vi "TestHemisphere.vi"() -> ()   [LabVIEW 2013]
uses:
  Data/TypeDefs/UTM Location.ctl
  <vilib>/myRIO/Common/Instrument Driver Framework/myRIO v1.0/UART/vis/myRIO v1.0 Close UART.vi
  <vilib>/myRIO/Common/Instrument Driver Framework/Utilities/vis/FPGA Ref Manager.vi
  <vilib>/myRIO/Common/Instrument Driver Framework/myRIO v1.0/myRIO v1.0 Reset FPGA.vi
  <vilib>/myRIO/Instrument Drivers/Utilities/Utilities.lvlib
panel:
  out "Serial Settings:Baud Rate":u32
  out "Raw string":string
  out "VISA read buffer":string
  out "Stop  Button\nHeartbeat":bool
  out "Stop Button\nLoop modulo":i32
  out "Read loop counter":i32
  out "Heartbeat":bool
  out "Roll":dbl
  out "Pitch":dbl
  out "Boat Speed":dbl
  out "Boat Direction":dbl
  out "Boat Location":T1 {"North" format="%#_10f"; "East" format="%#_8f"}
  in  "stop":bool
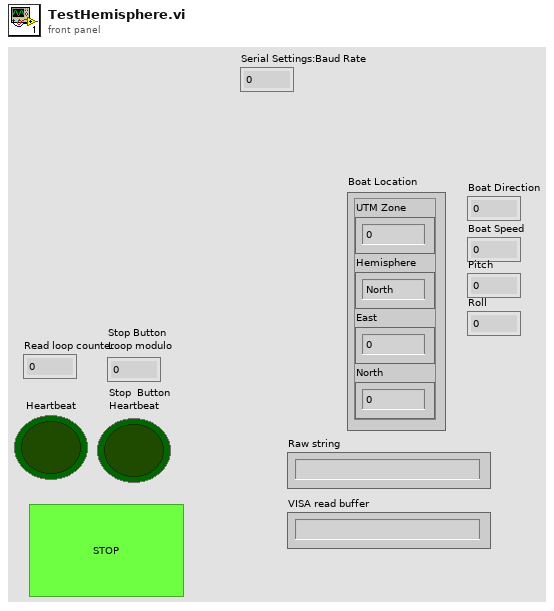
[diagram p1: front panel]
types:
  T1 = typedef "UTM Location.ctl" = cluster{"UTM Zone":dbl, "Hemisphere":enum16{"North", "South"}, "East":dbl, "North":dbl}
  T2 = typedef "Notifiers.ctl" = cluster{"BoatSpeed":refnum<notifier>, "WindSpeed":refnum<notifier>, "MissionCheckOff":refnum<notifier>, "EStop":refnum<notifier>, "SpeedOverWater":refnum<notifier>, "BoatDirection":refnum<notifier>, "Luffing":refnum<notifier>, "RudderForce":refnum<notifier>, "BatteryVoltage":refnum<notifier>, "StayForces":refnum<notifier>, "BoatLocation":refnum<notifier>, "Pitch":refnum<notifier>, "Roll":refnum<notifier>, "RateOfTurn":refnum<notifier>, "RelWindDirection":refnum<notifier>, "SailPositions":refnum<notifier>, "RudderPosition":refnum<notifier>, "IronsRange":refnum<notifier>, "AbsWindDirection":refnum<notifier>, "OverrideInformation":refnum<notifier>, "DynamixelTorques":refnum<notifier>, "MotorSetup":refnum<notifier>, "Airmar Status":refnum<notifier>, "HardwareOnline?":refnum<notifier>, "AcutalSimSailPositions":refnum<notifier>, "DynamixelCycleTracker":refnum<notifier>}
  T3 = typedef "GPS-Compass Queue Cluster.ctl" = cluster{"BoatLocation Queue":refnum<queue>, "BoatDirection Queue":refnum<queue>, "BoatSpeed Queue":refnum<queue>, "RateOfTurn Queue":refnum<queue>, "Pitch Queue":refnum<queue>, "Roll Queue":refnum<queue>}
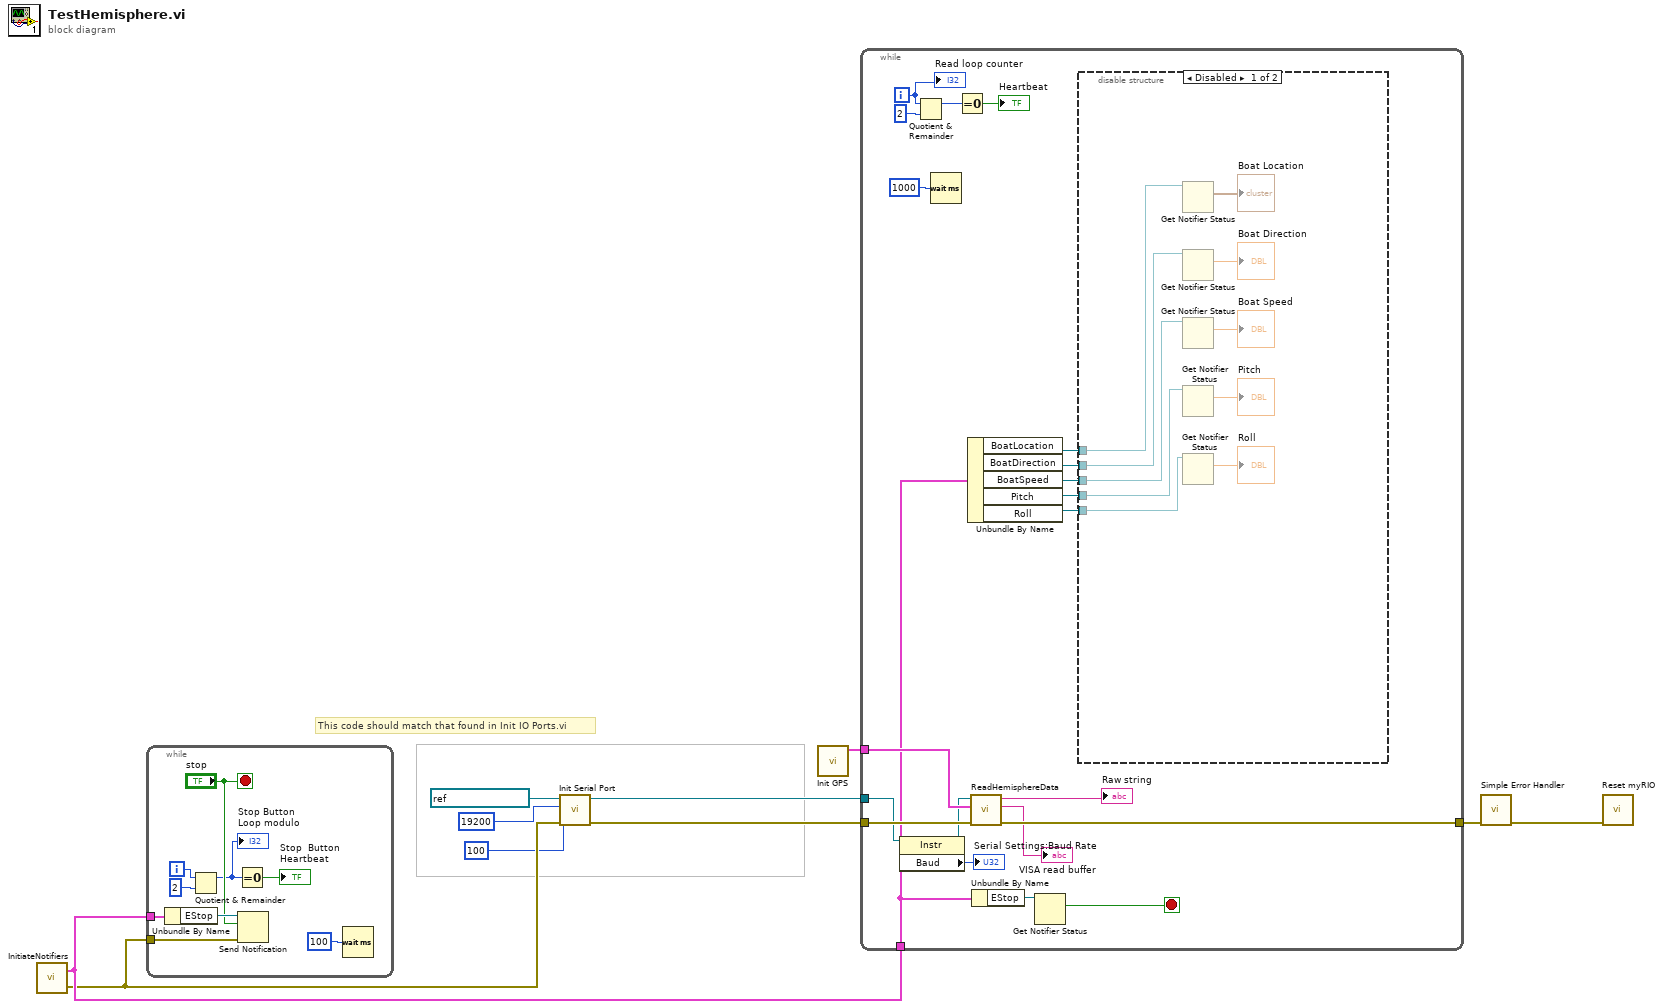
[diagram p0: block diagram]
diagram:
  # "This code should match that found in Init IO Ports.vi"
  n1 = call "InitiateNotifiers.vi"() -> ("error out"=w2:errorcluster, "NotifierReferences"=w7:T2)  [unwired: 2 in]
  n2 = while {
    tunnel: w7 -> [w17]
    tunnel: w2 -> [w11]
    i -> [w13]
    stop <- "stop" stop-if-true
    n3 = Unbundle By Name(w17) -> ("EStop"=w18:refnum<notifier>)
    n4 = Quotient & Remainder(x=w13, y=2) -> (x-y*floor(x/y)=w12:i32)  [unwired: 1 out]
    "Stop Button\nLoop modulo" <- w12
    n5 = Equal To 0?(x=w12) -> (x = 0?=→"Stop  Button\nHeartbeat":bool)
    n6 = Send Notification(notification="stop", notifier=w18, error in (no error)=w11) -> ()  [unwired: 2 out]
    n7 = Wait (ms)(milliseconds to wait=u32 100) -> ()  [unwired: 1 out]
  }
  n8 = call "Init Serial Port.vi"("error in (no error)"=w2, "Input\nbuffer size"=u32 100 ("Input\nbuffer size"), "baud rate"=u32 19200, "VISA Refnum in"=refnum<visa-resource-name> "ASRL1::INSTR") -> ("error out"=w5:errorcluster, "VISA Refnum out"=w6:refnum<visa-resource-name>)  [unwired: 6 in]
  n9 = call "Init GPS.vi"() -> ("GPS-Compass Queue Cluster"=w10:T3)  [unwired: 11 in]
  n10 = while {
    tunnel: w10 -> [w39]
    tunnel: w7 -> [w28]
    tunnel: [w31] -> w9
    tunnel: w6 -> [w23]
    tunnel: w5 -> [w29]
    i -> [w25]
    stop <- w20 stop-if-true
    n11 = property class="Instr"(reference=w23) -> (reference out=w22:refnum<visa-resource-name>, "Baud"=→"Serial Settings:Baud Rate":u32)  [unwired: 1 in, 1 out]
    n12 = Quotient & Remainder(x=w25, y=2) -> (x-y*floor(x/y)=w30:i32)  [unwired: 1 out]
    n13 = Wait (ms)(milliseconds to wait=u32 1000) -> ()  [unwired: 1 out]
    n14 = Equal To 0?(x=w30) -> (x = 0?=→"Heartbeat":bool)
    n15 = Unbundle By Name(w28) -> ("BoatLocation"=w38:refnum<notifier>, "BoatDirection"=w37:refnum<notifier>, "BoatSpeed"=w36:refnum<notifier>, "Pitch"=w35:refnum<notifier>, "Roll"=w34:refnum<notifier>)
    n16 = call "ReadHemisphereData.vi"("Error in"=w29, "Hemisphere Queue Cluster"=w39, "VISA UART port"=w22) -> ("Error out"=w31:errorcluster, "Sentence"=→"VISA read buffer":string, "Raw string"=→"Raw string":string)  [unwired: 6 in]
    n17 = Unbundle By Name(w28) -> ("EStop"=w27:refnum<notifier>)
    n18 = Get Notifier Status(notifier=w27) -> (current notification=w20:bool)  [unwired: 1 in, 4 out]
    n19 = disable-structure shown="Disabled" {
      disable-tunnel: w38 -> [w50 _]
      disable-tunnel: w37 -> [w49 _]
      disable-tunnel: w36 -> [w48 _]
      disable-tunnel: w35 -> [w47 _]
      disable-tunnel: w34 -> [w46 _]
      frame Disabled {
        n20 = Get Notifier Status(notifier=w50) -> (current notification=→"Boat Location":T1)  [unwired: 1 in, 4 out]
        n21 = Get Notifier Status(notifier=w49) -> (current notification=→"Boat Direction":dbl)  [unwired: 1 in, 4 out]
        n22 = Get Notifier Status(notifier=w48) -> (current notification=→"Boat Speed":dbl)  [unwired: 1 in, 4 out]
        n23 = Get Notifier Status(notifier=w47) -> (current notification=→"Pitch":dbl)  [unwired: 1 in, 4 out]
        n24 = Get Notifier Status(notifier=w46) -> (current notification=→"Roll":dbl)  [unwired: 1 in, 4 out]
      }
      frame Enabled {
      }
    }
    "Read loop counter" <- w25
  }
  n25 = call <vilib>:"Simple Error Handler.vi"("error in (no error)"=w9) -> ("error out"=w8:errorcluster)  [unwired: 4 in, 4 out]
  n26 = call <vilib>:"Reset myRIO.vi"("error in (no error)"=w8) -> ()  [unwired: 10 in, 1 out]
